vi "Write.vi"(8 "error in (no error)":errorcluster, 10 "Statement":T1={"timestamp"=timestamp(0 s since 1904-01-01), "level"=enum."INFO", "sourceTag"="", "originVI"="", "message"=""}, 11 "Appender in":refnum<class "Appender.lvclass">) -> (0 "error out":errorcluster, 3 "Appender out":refnum<class "Appender.lvclass">)   [LabVIEW 2026, in "Lumberjack.lvlib" / "Appender.lvclass"]
doc: "Deliver one accepted Statement to the sink. Called by HandleStatement after the statement passes the appender threshold and filter. Receives the structured Statement (not a formatted string): text sinks format via their own Layout here; the relay forwards or enqueues the Statement object. Abstract. DD, must override."
uses:
  Appender.lvclass
  TypeDefs/Statement.ctl
  TypeDefs/Severity.ctl
  Lumberjack.lvlib
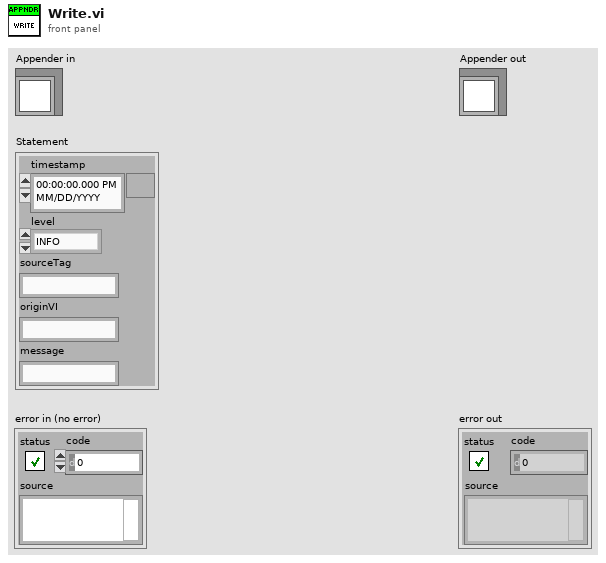
[diagram p1: front panel]
types:
  T1 = typedef "Lumberjack.lvlib/Statement.ctl" = cluster{"timestamp":timestamp, "level":T2, "sourceTag":string, "originVI":string, "message":string}
  T2 = typedef "Lumberjack.lvlib/Severity.ctl" = enum16{"OFF", "FATAL", "ERROR", "WARN", "INFO", "DEBUG", "TRACE", "ALL"}
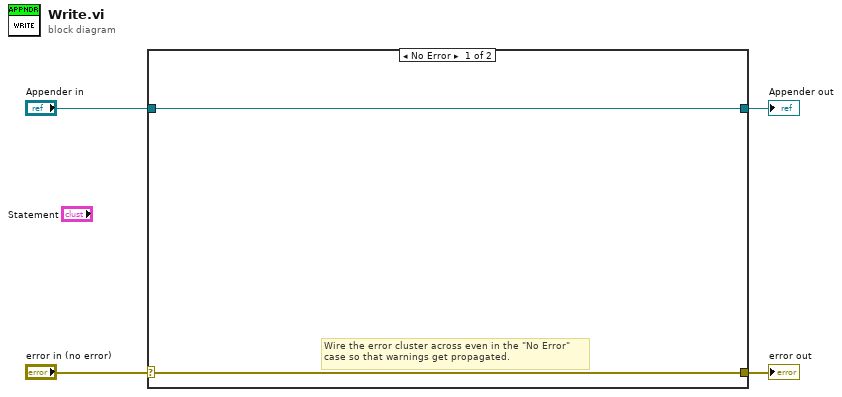
[diagram p0: block diagram]
diagram:
  n1 = case shown="No Error" "error in (no error)" {
    selector: "error in (no error)" -> [w5 w8]
    tunnel: [w5 w8] -> w3
    tunnel: [w6 w7] -> w1
    tunnel: "Appender in" -> [w6 w7]
    frame No Error {
      # "Wire the error cluster across even in the \"No Error\"\ncase so that warnings get propagated."
    }
    frame Error {
    }
  }
  "error out" <- w3
  "Appender out" <- w1
